vi "Generate Library HTML Documentation.vi"(4 "Root Folder Name":string="Toolkit", 6 "Requirement":string="Labstache", 7 "Destination":path=path "", 8 "Error In":errorcluster, 11 "Library File":path=path "") -> (0 "Error Out":errorcluster)   [LabVIEW 2018, in "Scripts.lvlib"]
uses:
  Scripts.lvlib
  Toolkit/Data/Map/Map.lvclass
  D:/Users/cfield/Code/Field R&D Services/Mustache/LabVIEW/trunk/src/Toolkit/Data/Datum/Datum.lvclass
  Toolkit/Data/Array/Array.lvclass
  Toolkit/Data/Map/Support/From String.vi
  Toolkit/Data/Map/Support/From Boolean.vi
  Toolkit/Data/Array/Support/From Data.vi
  Toolkit/Data/Map/Support/From Datum.vi
  Toolkit/Data/Map/Support/From Map Array.vi
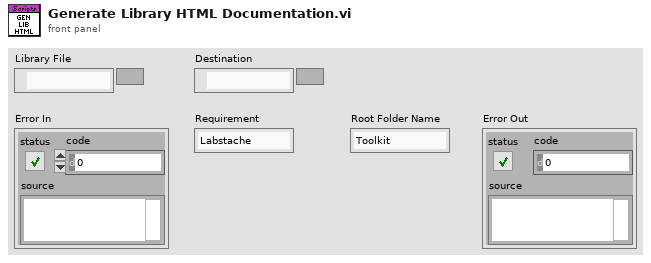
[diagram p1: front panel]
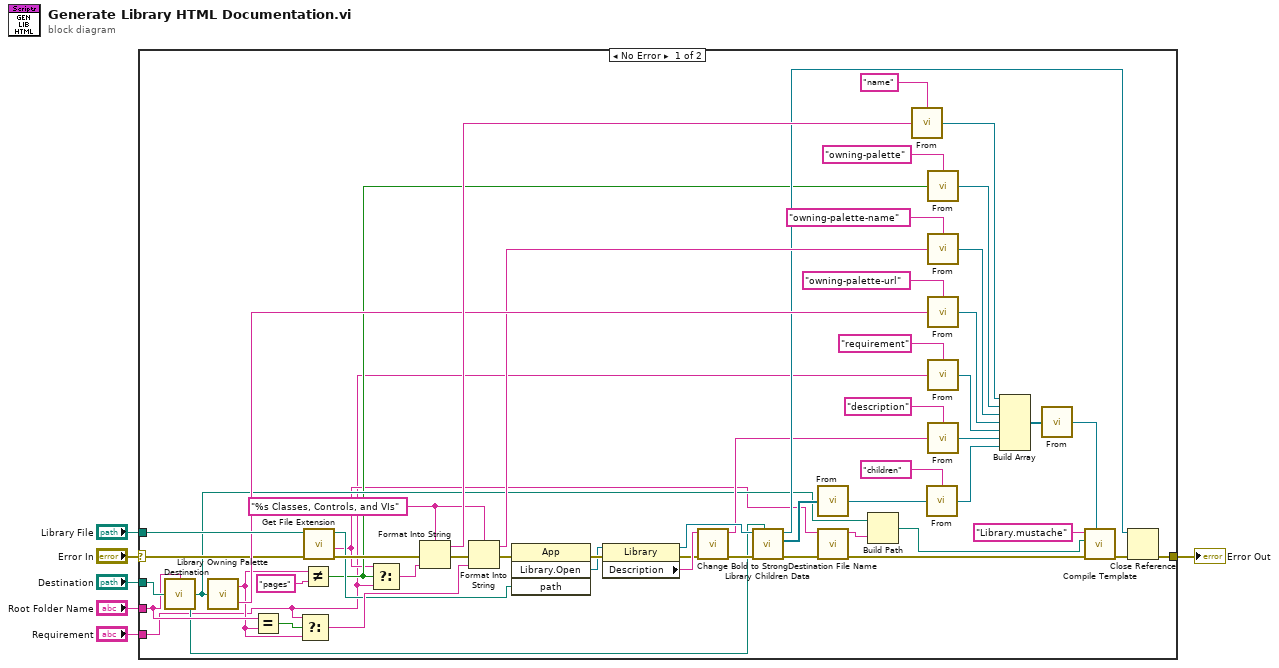
[diagram p0: block diagram]
diagram:
  n1 = case shown="No Error" "Error In" {
    selector: "Error In" -> [w33 w61]
    tunnel: "Destination" -> [w58 _]
    tunnel: "Library File" -> [w57 _]
    tunnel: [w38 w61] -> w5
    tunnel: "Root Folder Name" -> [w23 _]
    tunnel: "Requirement" -> [w7 _]
    frame No Error {
      w52 = "%s Classes, Controls, and VIs" ("format string")
      n2 = call "Destination.vi"("Root Destination In"=w58, "Root Folder Name"=w23) -> ("Root Destination Out"=w18:path)
      n3 = call "Library Owning Palette.vi"("Destination"=w18) -> ("Name"=w12:string, "URL"=w49:string)
      n4 = Equal?(x=w23, y=w12) -> (x = y?=w14:bool)
      n5 = Select(t=w7, s=w14, f=w12) -> (s? t:f=w43:string)
      n6 = Not Equal?(x=w12, y="pages") -> (x != y?=w10:bool)
      n7 = call <vilib>:"Get File Extension.vi"("error in (no error)"=w33, "file"=w57) -> ("error out"=w44:errorcluster, "filename without extension"=w9:string, "dup file"=w42:path)  [unwired: 5 in, 2 out]
      n8 = Select(t=w9, s=w10, f=w7) -> (s? t:f=w8:string)
      n9 = Format Into String(format string=w52, error in=w44, w8) -> (resulting string=w53:string, error out=w51:errorcluster)  [unwired: 1 in]
      n10 = Format Into String(format string=w52, error in=w51, w43) -> (resulting string=w46:string, error out=w45:errorcluster)  [unwired: 1 in]
      n11 = invoke class="App" method="Library.Open"(error in=w45, "path"=w42) -> (error out=w34:errorcluster, "Open Library"=w32:refnum<vi>)  [unwired: 2 in, 2 out]
      n12 = property class="Library"(reference=w32, error in=w34) -> (reference out=w36:refnum<vi>, error out=w20:errorcluster, "Description"=w22:string)
      n13 = call "Change Bold to Strong.vi"("Error In"=w20, "Bold Description"=w22) -> ("Error Out"=w19:errorcluster, "Strong Description"=w21:string)  [unwired: 8 in]
      n14 = call "Library Children Data.vi"("Destination"=w18, "Error In"=w19, "Library In"=w36) -> ("Error Out"=w28:errorcluster, "Array"=w27:refnum<class "Map.lvclass">[], "Library Out"=w29:refnum<vi>)  [unwired: 6 in]
      n15 = call-poly "From.vi"("Data"=w27) -> ("Array"=w26:refnum<class "Array.lvclass">)  [unwired: 1 in]
      n16 = call "Destination File Name.vi"("Error In"=w28, "File Stem"=w9) -> ("Error Out"=w39:errorcluster, "Destination File Name"=w40:string)  [unwired: 8 in]
      n17 = Build Path(base path=w18, name or relative path=w40) -> (appended path=w41:path)
      n18 = call-poly "From.vi"("Value"=w53, "Key"="name") -> ("Map"=w54:refnum<class "Map.lvclass">)
      n19 = call-poly "From.vi"("Value"=w26, "Key"="children") -> ("Map"=w24:refnum<class "Map.lvclass">)
      n20 = call-poly "From.vi"("Value"=w10, "Key"="owning-palette") -> ("Map"=w13:refnum<class "Map.lvclass">)
      n21 = call-poly "From.vi"("Value"=w46, "Key"="owning-palette-name") -> ("Map"=w55:refnum<class "Map.lvclass">)
      n22 = call-poly "From.vi"("Value"=w49, "Key"="owning-palette-url") -> ("Map"=w56:refnum<class "Map.lvclass">)
      n23 = call-poly "From.vi"("Value"=w7, "Key"="requirement") -> ("Map"=w16:refnum<class "Map.lvclass">)
      n24 = call-poly "From.vi"("Value"=w21, "Key"="description") -> ("Map"=w30:refnum<class "Map.lvclass">)
      n25 = Build Array(w54, w13, w55, w56, w16, w30, w24) -> (w59:refnum<class "Map.lvclass">[])
      n26 = call-poly "From.vi"("Maps"=w59) -> ("Map"=w60:refnum<class "Map.lvclass">)  [unwired: 1 in]
      n27 = call "Compile Template.vi"("Data"=w60, "Error In"=w39, "Output"=w41, "Template File Name"="Library.mustache" ("name or relative path")) -> ("Error Out"=w37:errorcluster)  [unwired: 7 in]
      n28 = Close Reference(reference=w29, error in (no error)=w37) -> (error out=w38:errorcluster)
    }
    frame Error {
    }
  }
  "Error Out" <- w5
